vi "DAQNavi Write (Analog 1D Wfm NChan NSamp).vi"(8 "error in (no error)":errorcluster, 9 "timeout":dbl=10.0, 10 "data":waveform(dbl)[](array[waveform]), 11 "task in":i32) -> (0 "error out":errorcluster, 2 "number of samples written per channel":u32, 3 "task out":i32)   [LabVIEW 2020]
uses:
  DAQNavi_LV.dll
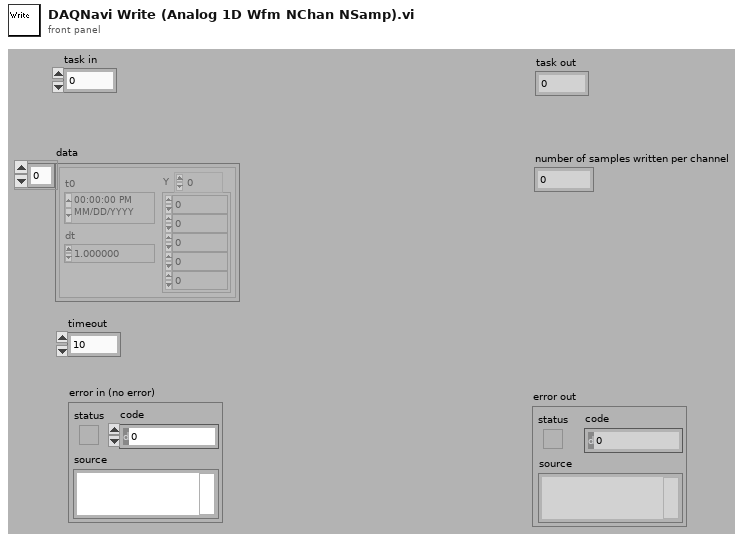
[diagram p1: front panel]
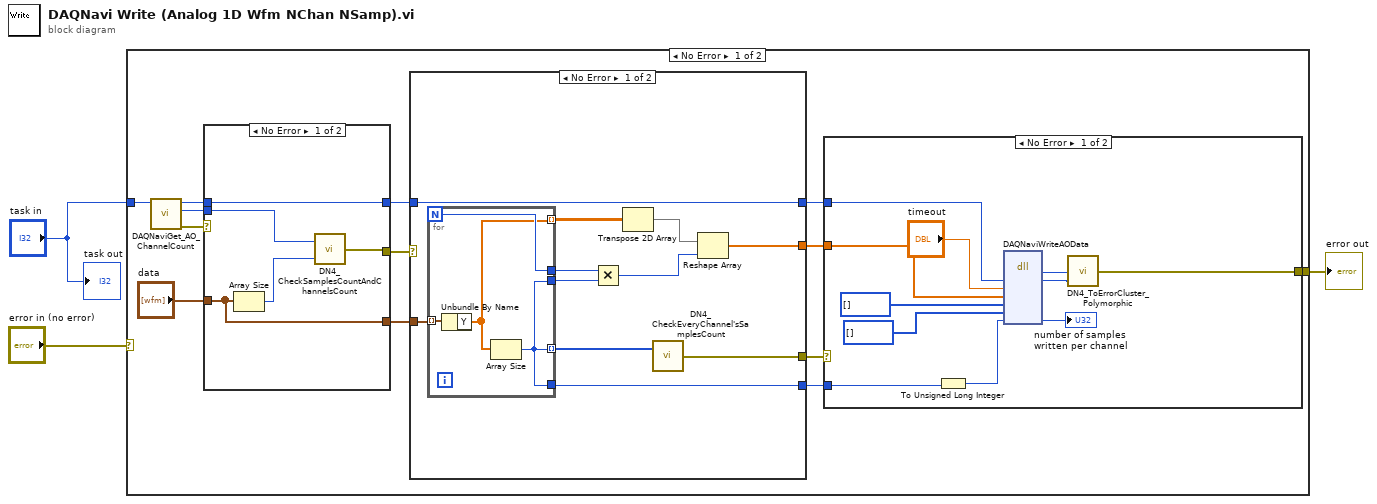
[diagram p0: block diagram]
diagram:
  n1 = case shown="No Error" "error in (no error)" {
    selector: "error in (no error)" -> [_ w54]
    tunnel: [w12 w54] -> w2
    tunnel: "task in" -> [w13 _]
    frame No Error {
      n2 = call "DAQNaviGet_AO_ChannelCount.vi"("task in"=w13) -> ("error out"=w16:errorcluster, "channel count"=w15:i32, "task out"=w14:i32)  [unwired: 1 in, 7 out]
      n3 = case shown="No Error" w16 {
        selector: w16 -> [_ w41]
        tunnel: w15 -> [w37 _]
        tunnel: [w35 w41] -> w11
        tunnel: [w38 w40] -> w8
        tunnel: w14 -> [w38 w40]
        tunnel: "data" -> [w34 w39]
        tunnel: [w34 w39] -> w10
        frame No Error {
          n4 = Array Size(array=w34) -> (size(s)=w36:i32)
          n5 = call "DN4_CheckSamplesCountAndChannelsCount.vi"("samples count"=w36, "channel count"=w37) -> ("error out"=w35:errorcluster)
        }
        frame Error {
        }
      }
      n6 = case shown="No Error" w11 {
        selector: w11 -> [_ w33]
        tunnel: w10 -> [w27 _]
        tunnel: [w18 w33] -> w9
        tunnel: [w23 w32] -> w7
        tunnel: w8 -> [w23 w32]
        tunnel: [w22 _] -> w6
        tunnel: [w17 _] -> w5
        frame No Error {
          n7 = for {
            N -> [w31]
            tunnel: w27 -> [w29] mode=indexing
            tunnel: [w30] -> w26 mode=indexing
            tunnel: [w28] -> w24 mode=indexing
            tunnel: [w30] -> w21
            tunnel: [w31] -> w20
            tunnel: [w30] -> w17
            n8 = Unbundle By Name(w29) -> ("Y"=w28:dbl[])
            n9 = Array Size(array=w28) -> (size(s)=w30:i32)
          }
          n10 = Multiply(x=w20, y=w21) -> (x*y=w19:i32)
          n11 = Transpose 2D Array(2D array=w24) -> (transposed array=w25:dbl[][])
          n12 = call "DN4_CheckEveryChannel'sSamplesCount.vi"("samples count"=w26) -> ("error out"=w18:errorcluster)  [unwired: 1 in]
          n13 = Reshape Array(w25, w19) -> (w22:dbl[])
        }
        frame Error {
        }
      }
      n14 = case shown="No Error" w9 {
        selector: w9 -> [_ w53]
        tunnel: [w52 w53] -> w12
        tunnel: w7 -> [w48 _]
        tunnel: w6 -> [w45 _]
        tunnel: w5 -> [w47 _]
        frame No Error {
          n15 = To Unsigned Long Integer(number=w47) -> (unsigned 32bit integer=w46:u32)
          n16 = dll-call lib="DAQNavi_LV.dll" fn="DAQNaviWriteAOData"("taskID"=w48, "timeout"="timeout", "scaledData"=w45, "rawData16"=u16[] [], "rawData32"=u32[] [], "samples"=w46) -> ("return type"=w49:i32, "taskID"=w42:i32, "samples"=→"number of samples written per channel":u32)  [unwired: 5 in, 4 out]
          n17 = call "DN4_ToErrorCluster_Polymorphic.vi"("task id"=w42, "error code"=w49) -> ("error out"=w52:errorcluster)  [unwired: 3 out]
        }
        frame Error {
        }
      }
    }
    frame Error {
    }
  }
  "error out" <- w2
  "task out" <- "task in"
